vi "decimateAllMatrix_mpc.vi"(8 "QP_params":T1={"maxIter"=0, "nuN"=24, "Ns_mpc"=0, "-beta"=-0.9987945556640625, "beta+1"=1.9987945556640625}, 10 "MPCRow (remainder)":dbl[](array[numeric])) -> (0 "MPC matrices":dbl[][](array[numeric]), 3 "MPCcol":dbl[](array[numeric]))   [LabVIEW 2017]
uses:
  fpga_VIs/fixed-point/single-axis/fxp_mpc/fgm_pipiline/quadProgParams_pipe.ctl
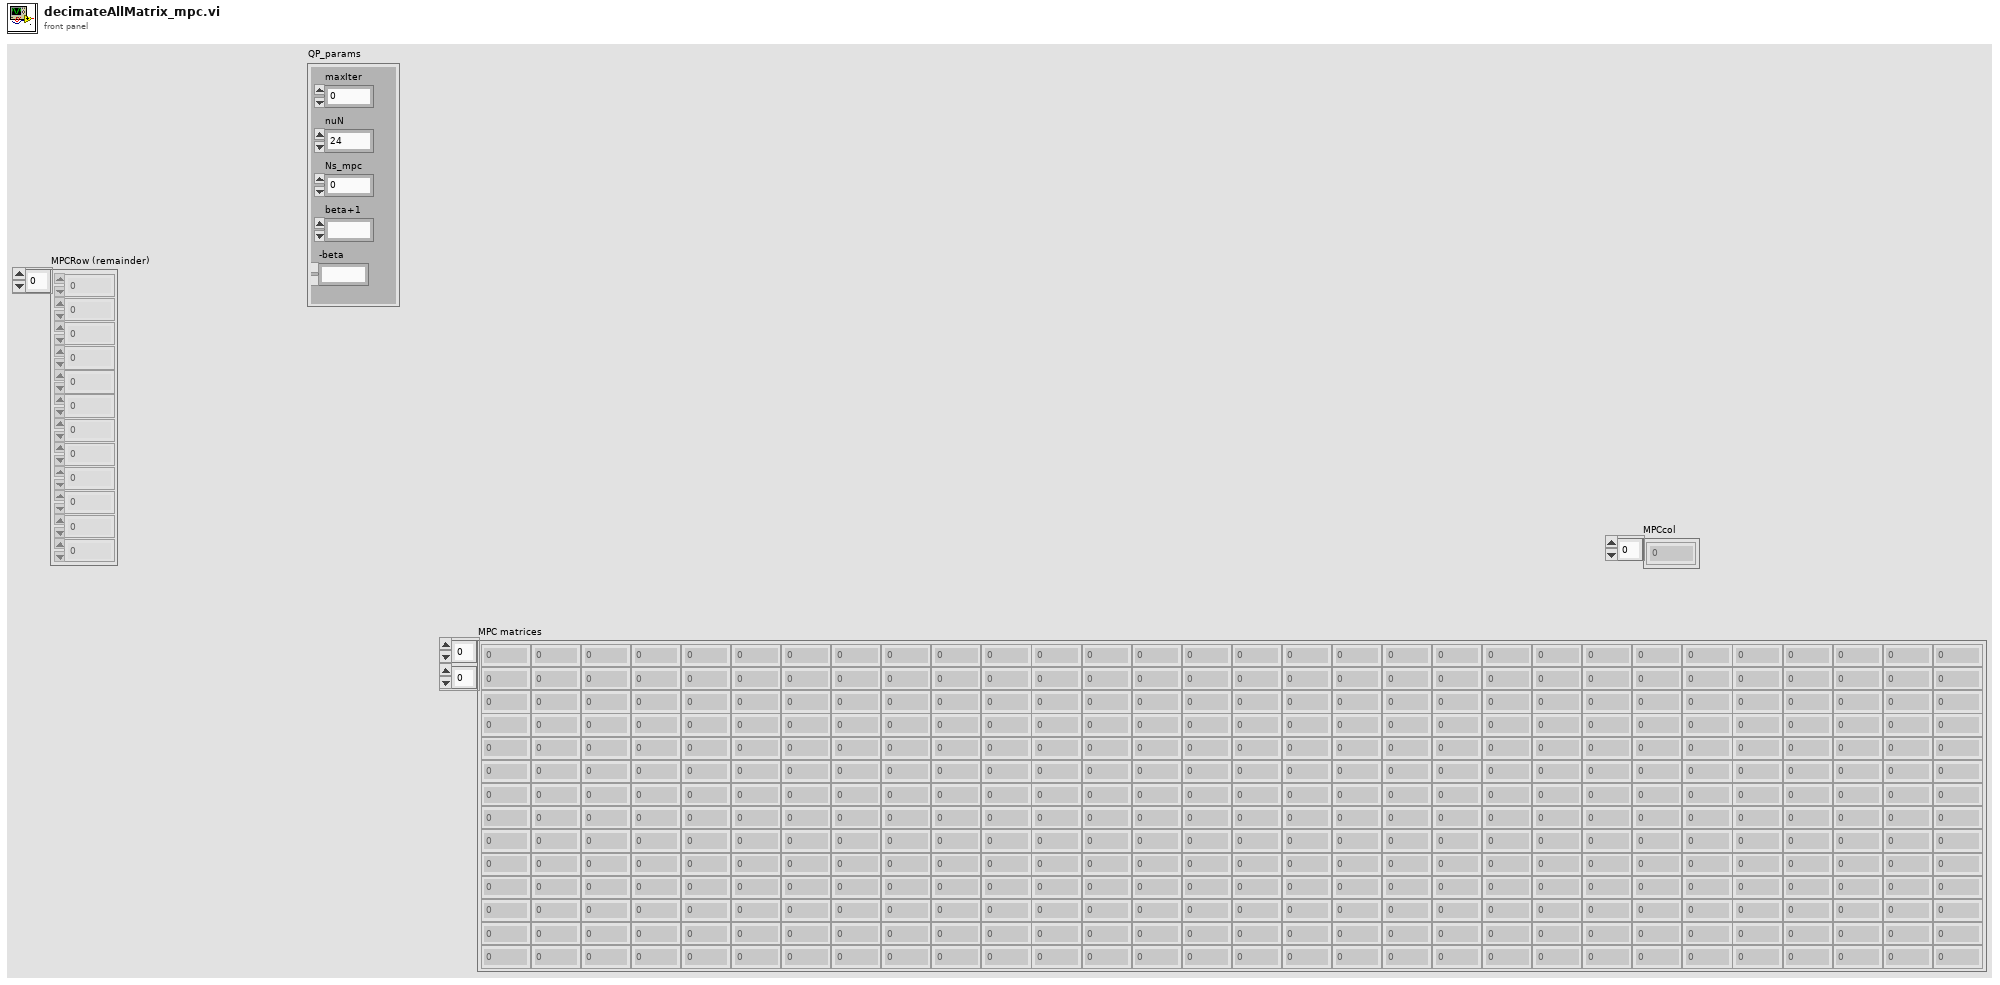
[diagram p1: front panel]
types:
  T1 = typedef "quadProgParams_pipe.ctl" = cluster{"maxIter":u16, "nuN":u16, "Ns_mpc":u16, "-beta":fxp<+/-,18,2>, "beta+1":fxp<+/-,18,2>}
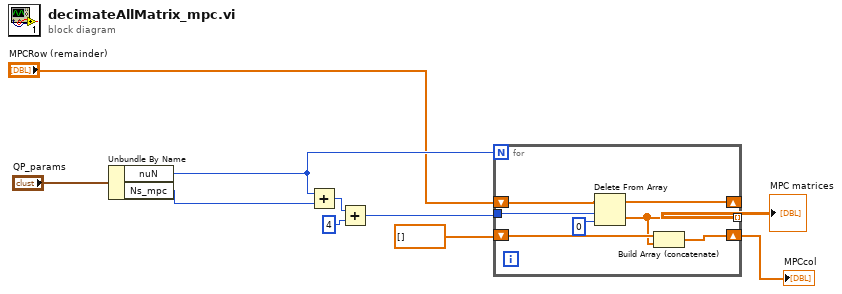
[diagram p0: block diagram]
diagram:
  n1 = Unbundle By Name("QP_params") -> ("nuN"=w4:u16, "Ns_mpc"=w5:u16)
  n2 = Add(x=w4, y=w5) -> (x+y=w10:u16)
  n3 = Add(x=w10, y=u16 4) -> (x+y=w8:u16)
  n4 = for {
    N: w4 -> [_]
    shift-right: [w14] -> _
    shift-left: "MPCRow (remainder)" -> [w16]
    tunnel: w8 -> [w15]
    tunnel: [w11] -> w7 mode=indexing
    shift-right: [w13] -> w2
    shift-left: dbl[] [] -> [w12]
    n5 = Delete From Array(array=w16, length=w15, index=0) -> (deleted portion=w11:dbl[], array with subset deleted=w14:dbl[])
    n6 = Build Array (concatenate)(w12, w11) -> (w13:dbl[])
  }
  "MPC matrices" <- w7
  "MPCcol" <- w2
